vi "Core.vi"(0 "Signal":T2, 5 "SwitchConfig":T3={"FreqCarrier"=0, "DeadtimeTicks"=1, "TriangleInc"=0.0}, 9 "enable":bool) -> (4 "SwitchPositions":T1, 15 "TriangleWave":fxp<+/-,32,4>)   [LabVIEW 2015, in "SPWM.lvlib"]
doc: "Sine PWM Algorithm\n\nThis algorithm is expected to be run in the LabVIEW FPGA inside a single cycle timed loop. It generates the on/off switch positions typically used with three-phase voltage source inverters. To configure this core use the SPWInterface.lvlib:CalcParams\n\nSignal - The signal we are trying to approximate with a sine PWM algorithm. Typically three sine waves with offset of 120 and -120 degrees is the input.\n\nSwitchConfig - Sets carrier frequency in ticks, deadtime in ticks, and the amount to increment the triangle per iteration."
uses:
  SPWM.lvlib
  SwitchConfig.ctl
  Signal.ctl
  SwitchPositions.ctl
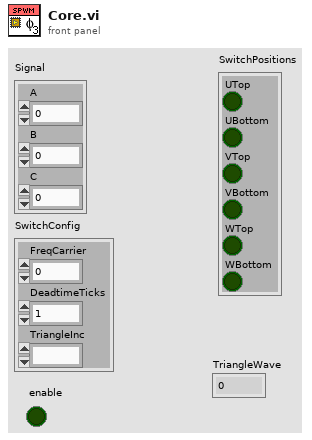
[diagram p1: front panel]
types:
  T1 = typedef "SPWM.lvlib/SwitchPositions.ctl" = cluster{"UTop":bool, "UBottom":bool, "VTop":bool, "VBottom":bool, "WTop":bool, "WBottom":bool}
  T2 = typedef "SPWM.lvlib/Signal.ctl" = cluster{"A":fxp<+/-,32,4>, "B":fxp<+/-,32,4>, "C":fxp<+/-,32,4>}
  T3 = typedef "SPWM.lvlib/SwitchConfig.ctl" = cluster{"FreqCarrier":u32, "DeadtimeTicks":u8, "TriangleInc":fxp<+/-,32,4>}
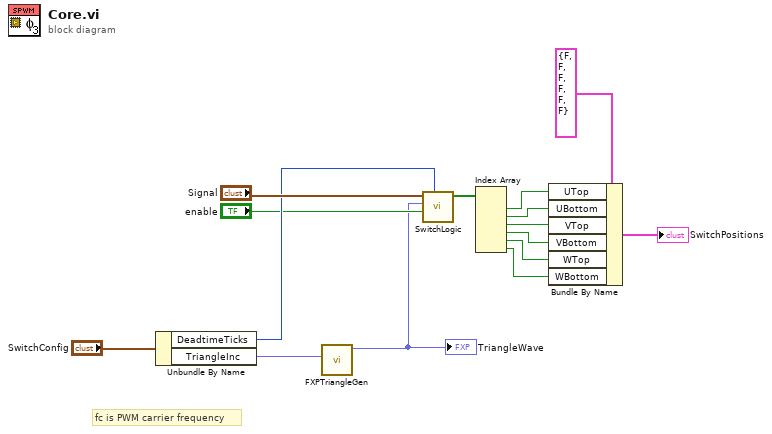
[diagram p0: block diagram]
diagram:
  # "fc is PWM carrier frequency"
  n1 = Unbundle By Name("SwitchConfig") -> ("DeadtimeTicks"=w5:u8, "TriangleInc"=w1:fxp<+/-,32,4>)
  n2 = call "FXPTriangleGen.vi"("triangleInc"=w1) -> ("triangle"=w2:fxp<+/-,32,4>)  [unwired: 10 in]
  "TriangleWave" <- w2
  n3 = call "SwitchLogic.vi"("Deadtime"=w5, "enable"="enable", "triangle"=w2, "sine waves"="Signal") -> ("switch values"=w4:bool[])  [unwired: 7 in]
  n4 = Index Array(array=w4) -> (element #1=w15:bool, element #2=w14:bool, element #3=w13:bool, element #4=w12:bool, element #5=w11:bool, element #6=w10:bool)  [unwired: 6 in]
  n5 = Bundle By Name(cluster=T1 {"UTop"=FALSE, "UBottom"=FALSE, "VTop"=FALSE, "VBottom"=FALSE, "WTop"=FALSE, "WBottom"=FALSE} ("SwitchPositions"), "UTop"=w15, "UBottom"=w14, "VTop"=w13, "VBottom"=w12, "WTop"=w11, "WBottom"=w10) -> (→"SwitchPositions":T1)
